vi "Remove State from Routing Channel.vi"(8 "error in (no error)":errorcluster, 10 "State":string, 11 "Channel Ref in":T1 format="%.0x") -> (0 "error out":errorcluster, 3 "Channel Ref out":T1=18446744073709551615 format="%.0x")   [LabVIEW 2017, in "SLSC Switch Scripting.lvlib"]
uses:
  SLSC Switch Scripting.lvlib
  <vilib>/NI Veristand/Custom Device API/Custom Device Item Ref.ctl
  <vilib>/NI VeriStand/Custom Device API/Custom Device API.lvlib
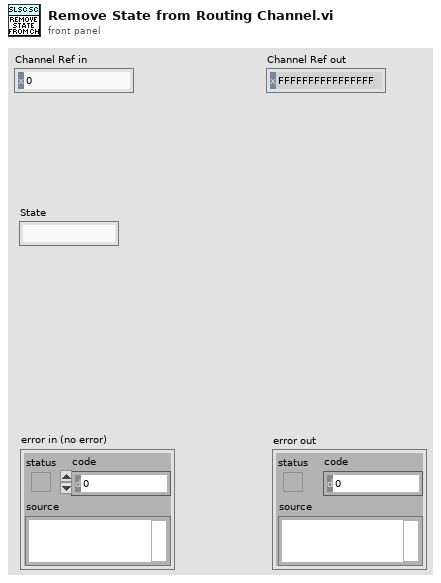
[diagram p1: front panel]
types:
  T1 = typedef "Custom Device API.lvlib/Custom Device Item Ref.ctl" = u64
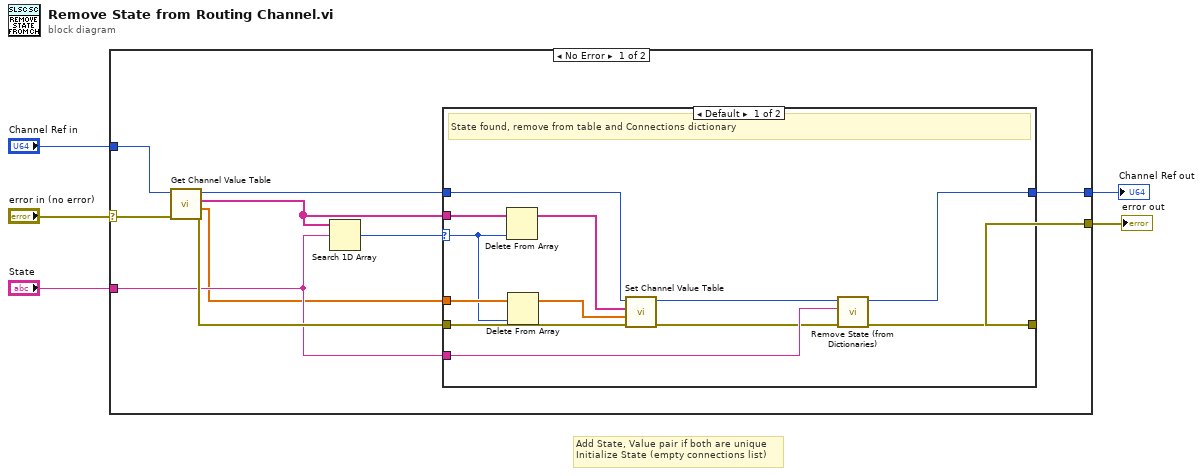
[diagram p0: block diagram]
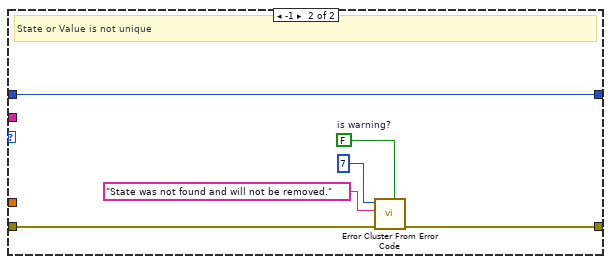
[diagram p2: hidden frame]
diagram:
  # "Add State, Value pair if both are unique\nInitialize State (empty connections list)"
  n1 = case shown="No Error" "error in (no error)" {
    selector: "error in (no error)" -> [w14 w35]
    tunnel: [w10 w35] -> w1
    tunnel: "Channel Ref in" -> [w15 w34]
    tunnel: [w11 w34] -> w3
    tunnel: "State" -> [w8 _]
    frame No Error {
      n2 = call "Get Channel Value Table.vi"("error in (no error)"=w14, "Channel Ref in"=w15) -> ("error out"=w12:errorcluster, "Values"=w7:dbl[], "States"=w9:string[], "Channel Ref out"=w13:T1)  [unwired: 6 in]
      n3 = Search 1D Array(1D array=w9, element=w8) -> (index of element=w6:i32)  [unwired: 1 in]
      n4 = case shown="Default" w6 {
        selector: w6 -> [w18 _]
        tunnel: w13 -> [w27 w28]
        tunnel: w12 -> [w26 w30]
        tunnel: w7 -> [w19 _]
        tunnel: [w24 w28] -> w11
        tunnel: [w21 w29] -> w10
        tunnel: w9 -> [w20 _]
        tunnel: w8 -> [w23 _]
        frame Default {
          # "State found, remove from table and Connections dictionary"
          n5 = Delete From Array(array=w20, index=w18) -> (array with subset deleted=w16:string[])  [unwired: 1 in, 1 out]
          n6 = Delete From Array(array=w19, index=w18) -> (array with subset deleted=w17:dbl[])  [unwired: 1 in, 1 out]
          n7 = call "Set Channel Value Table.vi"("error in (no error)"=w26, "Values"=w17, "States"=w16, "Channel Ref in"=w27) -> ("error out"=w22:errorcluster, "Channel Ref out"=w25:T1)  [unwired: 6 in]
          n8 = call "Remove State (from Dictionaries).vi"("error in (no error)"=w22, "State"=w23, "Channel Ref in"=w25) -> ("error out"=w21:errorcluster, "Channel Ref out"=w24:T1)  [unwired: 7 in]
        }
        frame -1 {
          w32 = FALSE  # is warning?
          # "State or Value is not unique"
          n9 = call <vilib>:"Error Cluster From Error Code.vi"("is warning? (False)"=w32, "error in (no error)"=w30, "error message (\"\")"="State was not found and will not be removed." ("error message (\"\")"), "error code (0)"=7) -> ("error out"=w29:errorcluster)  [unwired: 5 in]
        }
      }
    }
    frame Error {
    }
  }
  "Channel Ref out" <- w3
  "error out" <- w1
